vi "Authentication.vi"(8 "error in (no error)":errorcluster, 10 "Authentication":string, 11 "Identify in":refnum<class "Identify.lvclass">) -> (0 "error out":errorcluster, 3 "Identify out":refnum<class "Identify.lvclass">)   [LabVIEW 2020, in "obs-websocket.lvlib" / "Identify.lvclass"]
uses:
  Identify.lvclass
  Identify.lvclass/Identify.ctl
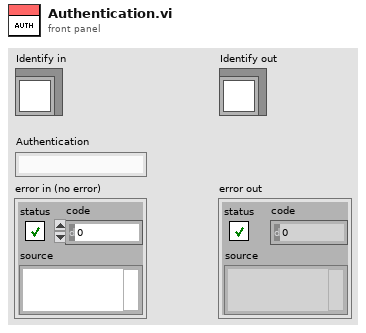
[diagram p1: front panel]
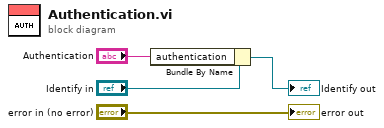
[diagram p0: block diagram]
diagram:
  n1 = Bundle By Name(cluster="Identify in", "authentication"="Authentication") -> (→"Identify out":refnum<class "Identify.lvclass">)
  "error out" <- "error in (no error)"
